vi "Initial Matrix (DBL).vi"(10 "column":i32, 11 "row":i32) -> (0 "error":i32, 3 "Matrix":T1)   [LabVIEW 2020, in "NI_AALBase.lvlib"]
uses:
  NI_AALBase.lvlib
  RealMatrix.ctl
  <resource>/lvanlys.dll
  NI_Matrix.lvlib
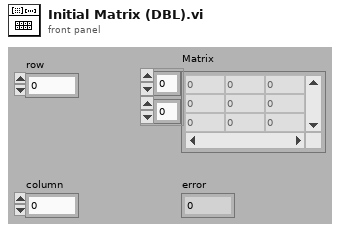
[diagram p1: front panel]
types:
  T1 = typedef "NI_Matrix.lvlib/RealMatrix.ctl" = dbl[][]
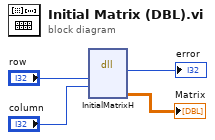
[diagram p0: block diagram]
diagram:
  n1 = dll-call lib="C:/Program Files (x86)/National Instruments/LabVIEW 2020/resource/lvanlys.*" fn="InitialMatrixH"("row"="row", "col"="column") -> (→"error":i32, "xH"=→"Matrix":dbl[][])  [unwired: 6 in, 2 out]
